vi "TW Update Missing Paths.vi"(8 "error in (no error)":errorcluster, 9 "New Subname":string, 10 "Subname to Replace":string, 11 "GObject in":refnum<vi>) -> (0 "error out":errorcluster)   [LabVIEW 2021, in "LV Scripting Utilities.lvlib"]
uses:
  LV Scripting Utilities.lvlib
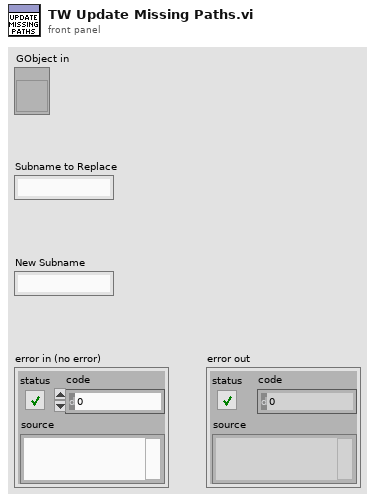
[diagram p1: front panel]
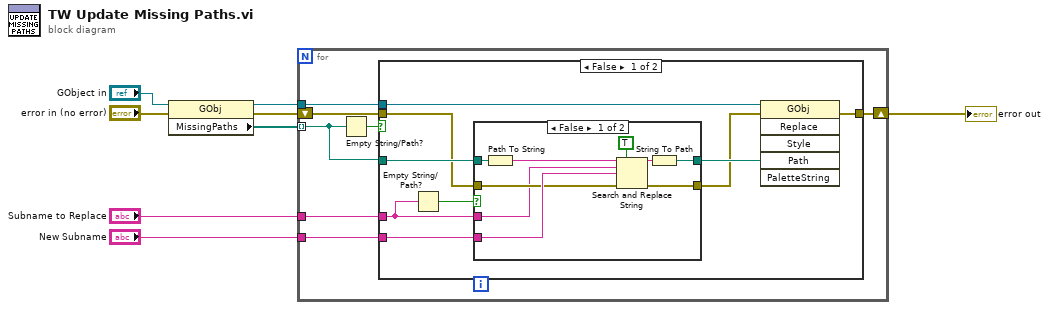
[diagram p0: block diagram]
diagram:
  n1 = property class="GObj"(reference="GObject in", error in="error in (no error)") -> (reference out=w1:refnum<vi>, error out=w3:errorcluster, "MissingPaths"=w2:path[])
  n2 = for {
    tunnel: w1 -> [w15]
    tunnel: w2 -> [w13] mode=indexing
    shift-right: [w11] -> w6
    shift-left: w3 -> [w12]
    tunnel: "Subname to Replace" -> [w10]
    tunnel: "New Subname" -> [w9]
    n3 = Empty String/Path?(string/path=w13) -> (empty?=w14:bool)
    n4 = case shown="False" w14 {
      tunnel: w15 -> [w24 _]
      tunnel: w13 -> [w22 _]
      tunnel: w12 -> [w19 w36]
      tunnel: [w23 w36] -> w11
      tunnel: w10 -> [w17 _]
      tunnel: w9 -> [w20 _]
      frame False {
        n5 = Empty String/Path?(string/path=w17) -> (empty?=w16:bool)
        n6 = case shown="False" w16 {
          tunnel: w22 -> [w30 w35]
          tunnel: [w29 w35] -> w21
          tunnel: w20 -> [w28 _]
          tunnel: w19 -> [w27 w34]
          tunnel: [w26 w34] -> w18
          tunnel: w17 -> [w25 _]
          frame False {
            n7 = Path To String(path=w30) -> (string=w31:string)
            n8 = Search and Replace String(replace all?=TRUE ("replace all? (F)"), input string=w31, search string=w25, replace string=w28, error in=w27) -> (result string=w32:string, error out=w26:errorcluster)  [unwired: 3 in, 2 out]
            n9 = String To Path(string=w32) -> (path=w29:path)
          }
          frame True {
          }
        }
        n10 = invoke class="GObj" method="Replace"(reference=w24, error in=w18, "Path"=w21) -> (error out=w23:errorcluster)  [unwired: 3 in, 5 out]
      }
      frame True {
      }
    }
  }
  "error out" <- w6
